vi "create_submenu_item.vi"(7 "SubMenu Title":string, 8 "error in (no error)":errorcluster, 9 "lookup string":string, 10 "MenuItem references":refnum<k24>[](array[refnum]), 11 "BalloonNotifier in":refnum<class "BalloonNotifier.lvclass">) -> (0 "error out":errorcluster, 2 "SubMenuItem reference":refnum<k24>, 3 "BalloonNotifier out":refnum<class "BalloonNotifier.lvclass">)   [LabVIEW 2010, in "BalloonNotifier.lvclass"]
uses:
  BalloonNotifier.lvclass
  System.Windows.Forms
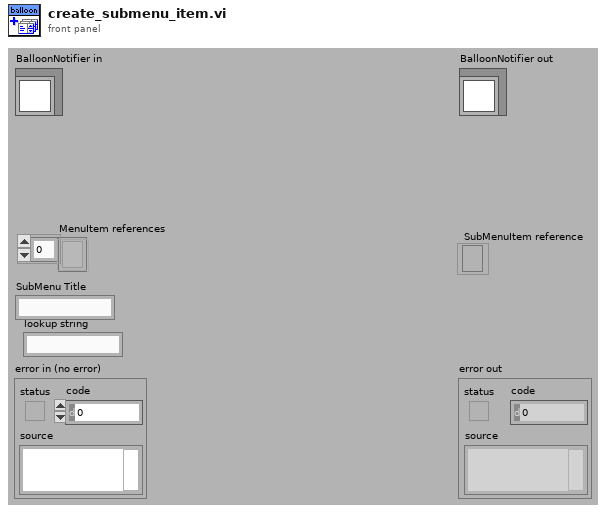
[diagram p1: front panel]
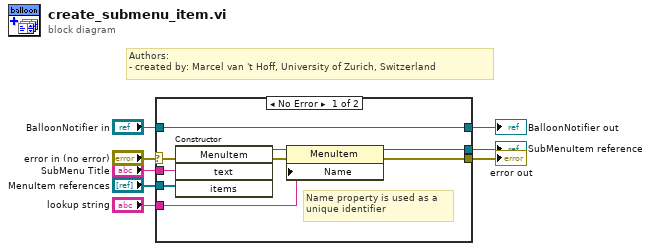
[diagram p0: block diagram]
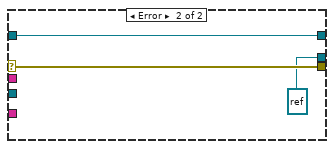
[diagram p2: hidden frame]
diagram:
  # "Authors: \n- created by: Marcel van 't Hoff, University of Zurich, Switzerland"
  n1 = case shown="No Error" "error in (no error)" {
    selector: "error in (no error)" -> [w10 w20]
    tunnel: "MenuItem references" -> [w17 _]
    tunnel: [w15 refnum<k24> refnum ("new reference")] -> w1
    tunnel: [w13 w20] -> w7
    tunnel: "SubMenu Title" -> [w12 _]
    tunnel: "lookup string" -> [w11 _]
    tunnel: [w9 w18] -> w3
    tunnel: "BalloonNotifier in" -> [w9 w18]
    frame No Error {
      # "Name property is used as a \nunique identifier"
      n2 = constructor class="MenuItem"(error in=w10, "text"=w12, "items"=w17) -> (reference out=w16:refnum<k24>, error out=w14:errorcluster)  [unwired: 2 in, 3 out]
      n3 = property class="MenuItem"(reference=w16, error in=w14, "Name"=w11) -> (reference out=w15:refnum<k24>, error out=w13:errorcluster)
    }
    frame Error {
    }
  }
  "error out" <- w7
  "BalloonNotifier out" <- w3
  "SubMenuItem reference" <- w1
